vi "BattlesonEXC3tsk4.vi"() -> ()   [LabVIEW 2014, in "Battleson_Robot_12-2-16.lvrbt"]
uses:
  C:/Users/blb1094/Documents/LabVIEW Data/NXTRobotics/Projects/Battleson_Robot_12-2-16/Battleson_Robot_12-2-16.lvrbt
panel:
  out "XY Graph":cluster{"X":dbl, "Y":dbl}[](graph)
  out "Waveform Graph":dbl[](graph)
  out "Sweep Chart":cluster{dbl, dbl}(graph)
  out "Scope Chart":cluster{dbl, dbl}(graph)
  out "Strip Chart":cluster{dbl, dbl}(graph)
  in  "stop":bool
  out "Moving Average":dbl
  out "Random Number":dbl
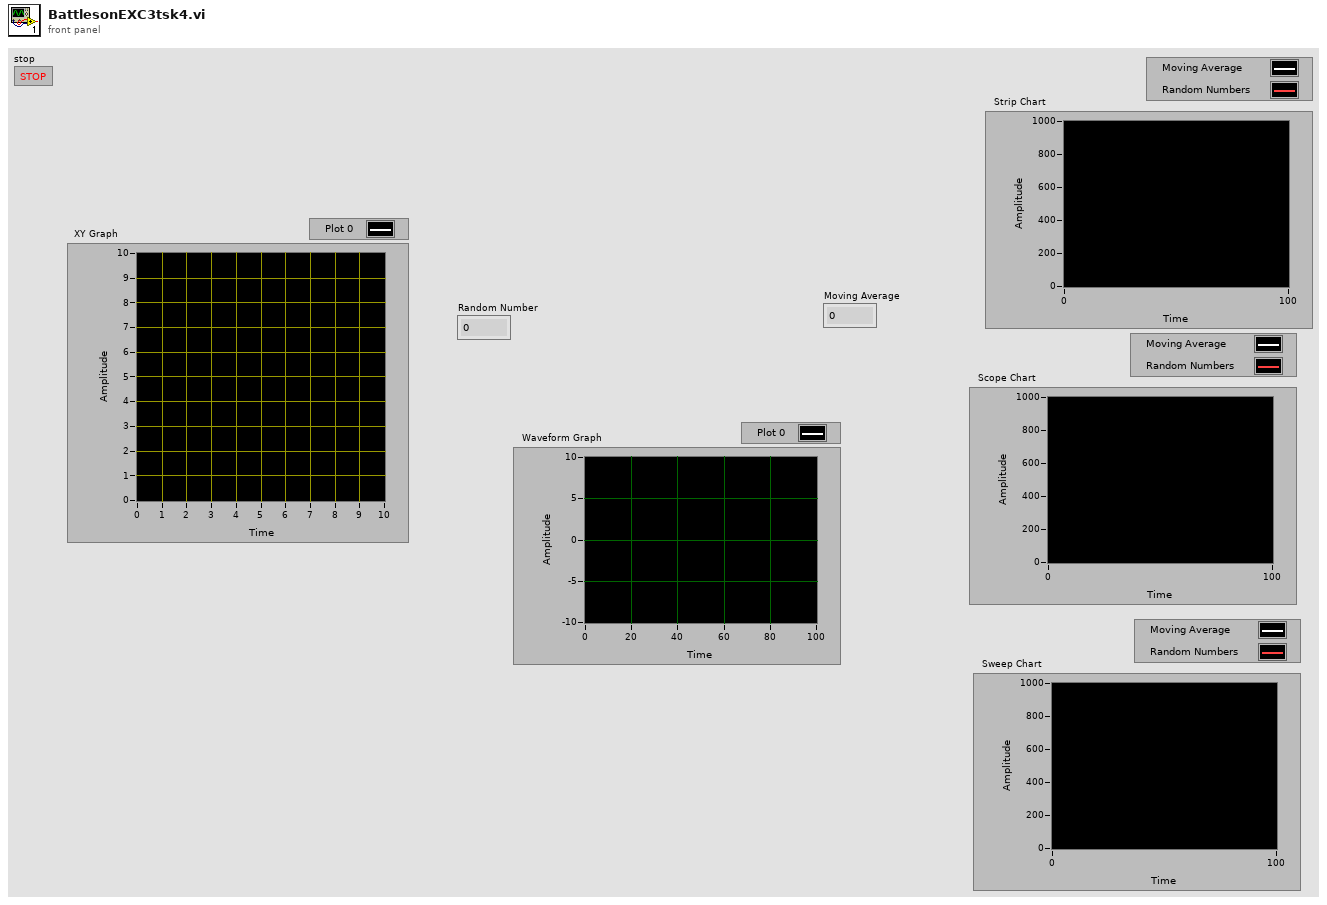
[diagram p1: front panel]
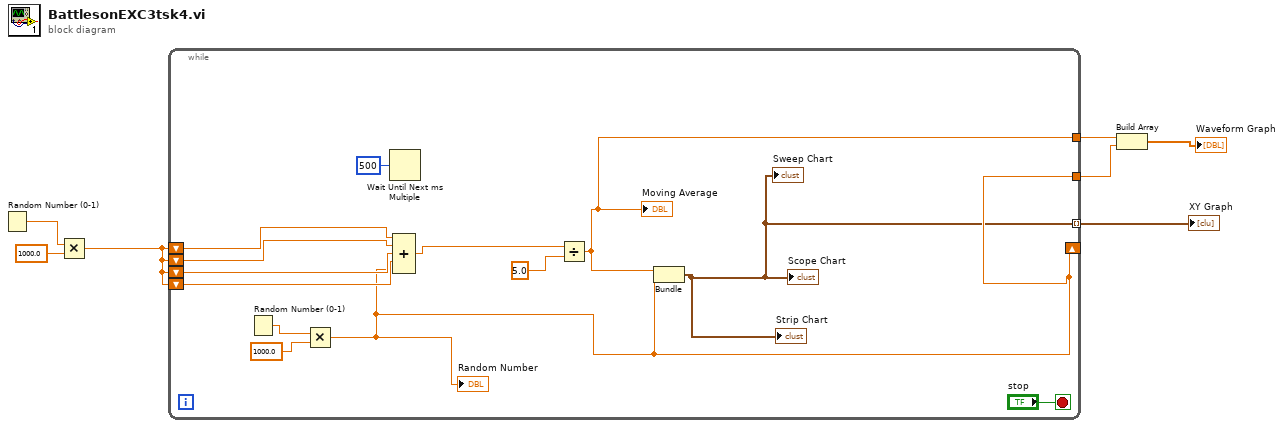
[diagram p0: block diagram]
diagram:
  n1 = Random Number (0-1)() -> (number: 0 to 1=w7:dbl)
  n2 = Multiply(x=w7, y=1000.0) -> (x*y=w5:dbl)
  n3 = while {
    shift-right: [w9] -> _
    shift-left: w5 -> [w15]
    shift-left: w5 -> [w17]
    shift-left: w5 -> [w18]
    shift-left: w5 -> [w16]
    tunnel: [w10] -> w3
    tunnel: [w9] -> w2
    tunnel: [w8] -> w1 mode=indexing
    stop <- "stop" stop-if-true
    n4 = Random Number (0-1)() -> (number: 0 to 1=w20:dbl)
    n5 = Multiply(x=w20, y=1000.0) -> (x*y=w9:dbl)
    "Random Number" <- w9
    n6 = Wait Until Next ms Multiple(millisecond multiple=u32 500) -> ()  [unwired: 1 out]
    n7 = Compound Arithmetic op=ADD(w15, w16, w17, w18, w9) -> (w14:dbl)
    n8 = Divide(x=w14, y=5.0) -> (x/y=w10:dbl)
    "Moving Average" <- w10
    n9 = Bundle(w10, w9) -> (w8:cluster{dbl, dbl})  [unwired: 1 in]
    "Strip Chart" <- w8
    "Scope Chart" <- w8
    "Sweep Chart" <- w8
  }
  "XY Graph" <- w1
  n10 = Build Array(w3, w2) -> (→"Waveform Graph":dbl[])
